vi "Parameter.vi"(8 "error in":errorcluster, 11 "Node Ptr":T1 format="%.0x") -> (0 "error out":errorcluster)   [LabVIEW 2020, in "Ballard MIL-STD-1553 System Explorer.lvlib" / "Implementation.lvlib"]
uses:
  Implementation.lvlib
  <vilib>/NI VeriStand/Custom Device API/Custom Device Item Ref.ctl
  <vilib>/NI VeriStand/Custom Device API/Custom Device API.lvlib
  Scripting/Ballard MIL-STD-1553 Scripting.lvlib
panel:
  out "Encoding Type":enum16{"BNR", "BCD", "Discrete"}(ring)
  out "Unit":string
  out "Scale Offset":dbl
  out "Scale Factor":dbl=1.0
  out "Signed?":bool=TRUE
  out "Number of Bits":i32=16
  out "Start Bit":i32
  out "default value":dbl caption="Default Value (Scaled)"
  in  "SHDocVw.IWebBrowser":refnum<k7>(container)
  in  "General Header":cluster{"Section Name":string}={"Section Name"="Ballard MIL-STD-1553 - Parameter"}
  in  "Description":string
  out "Name":string
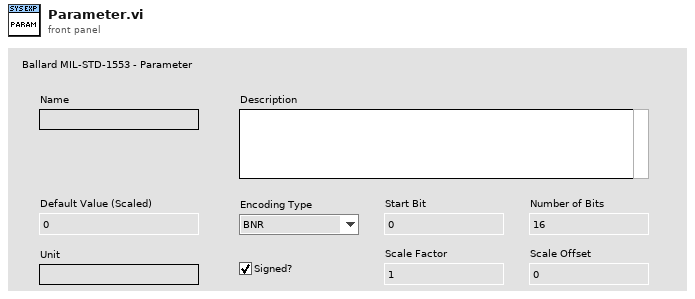
[diagram p1: front panel]
types:
  T1 = typedef "Custom Device API.lvlib/Custom Device Item Ref.ctl" = u64
  T2 = typedef "Custom Device API.lvlib/Custom Device Channel.ctl" = cluster{"Type":T3, "Units":string, "Default Value":dbl, "Faultable":bool, "Scalable":bool}
  T3 = typedef "Custom Device API.lvlib/Custom Device Channel Type.ctl" = enum16{"Input", "Output"}
  T4 = typedef "Parameter Definition.ctl" = cluster{"start index":i32, "size (bits)":i32, "encoding":enum16{"BNR", "BCD", "Discrete"}, "signed":bool, "multiplier":dbl, "offset":dbl}
  T5 = typedef "Custom Device API.lvlib/Custom Device Commands.ctl" = enum16{"Default", "Item renamed", "Shutdown", "Dynamic button pressed"}
  T6 = typedef "Custom Device API.lvlib/Custom Device Item Info.ctl" = cluster{"Name":string, "Is Channel":bool, "GUID":string, "Is Waveform":bool}
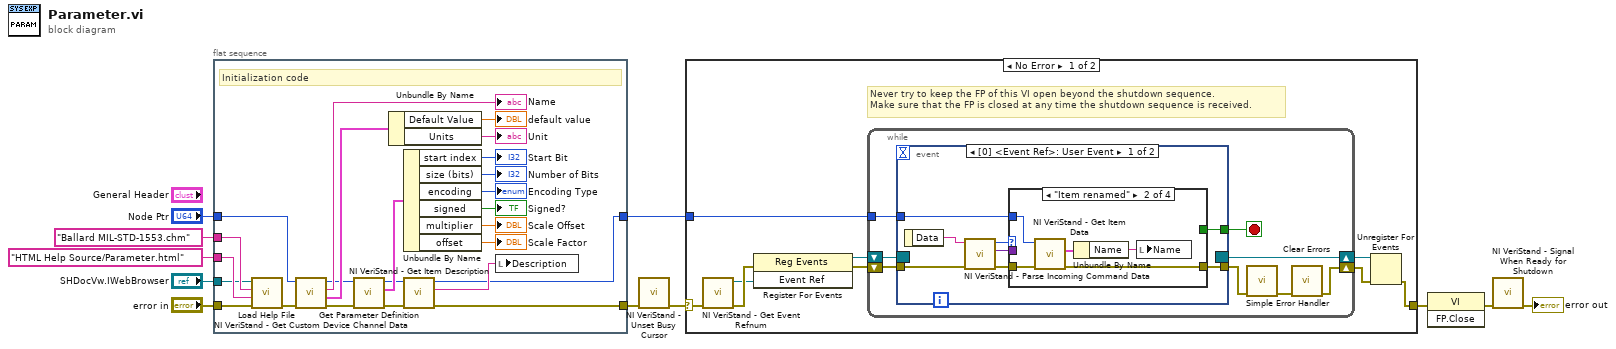
[diagram p0: block diagram]
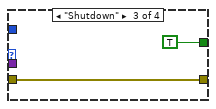
[diagram p3: hidden frame]
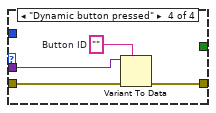
[diagram p4: hidden frame]
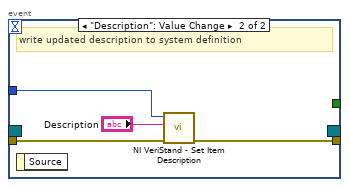
[diagram p5: hidden frame]
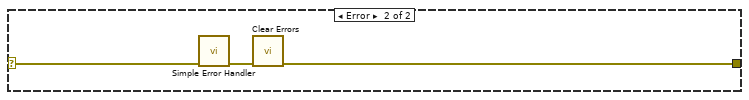
[diagram p6: hidden frame]
diagram:
  n1 = flat-sequence "Initialization code" {
    tunnel: "error in" -> [w34]
    tunnel: "Node Ptr" -> [w30]
    tunnel: [w13] -> w7
    tunnel: [w12] -> w4
    tunnel: "SHDocVw.IWebBrowser" -> [w31]
    tunnel: "HTML Help Source/Parameter.html" ("CD_CHM_Section") -> [w33]
    tunnel: "Ballard MIL-STD-1553.chm" ("CD_CHM_FileName") -> [w32]
    frame #0 {
      # "Initialization code"
      n2 = call "Load Help File.vi"("error in (no error)"=w34, "HTML File to Load"=w33, "Main CHM File"=w32, "Browser"=w31) -> ("error out"=w28:errorcluster)  [unwired: 7 in]
      n3 = call <vilib>:"NI VeriStand - Get Custom Device Channel Data.vi"("error in (no error)"=w28, "Channel Ref in"=w30) -> ("error out"=w16:errorcluster, "Channel"=w29:T2, "Channel Name"=→"Name":string, "Channel Ref out"=w17:T1)  [unwired: 4 in, 2 out]
      n4 = call "Get Parameter Definition.vi"("error in"=w16, "parameter in"=w17) -> ("error out"=w14:errorcluster, "parameter definition"=w24:T4, "parameter out"=w15:T1)  [unwired: 7 in]
      n5 = Unbundle By Name(w29) -> ("Default Value"=→"default value":dbl, "Units"=→"Unit":string)
      n6 = Unbundle By Name(w24) -> ("start index"=→"Start Bit":i32, "size (bits)"=→"Number of Bits":i32, "encoding"=→"Encoding Type":enum16{"BNR", "BCD", "Discrete"}, "signed"=→"Signed?":bool, "multiplier"=→"Scale Offset":dbl, "offset"=→"Scale Factor":dbl)
      n7 = call <vilib>:"NI VeriStand - Get Item Description.vi"("error in (no error)"=w14, "Item Ref in"=w15) -> ("error out"=w13:errorcluster, "Description"=w35:string, "Item Ref out"=w12:T1)  [unwired: 7 out]
      n8 = local write "Description"(w35) -> ()
    }
  }
  n9 = call <vilib>:"NI VeriStand - Unset Busy Cursor.vi"("error in (no error)"=w7) -> ("error out"=w6:errorcluster)  [unwired: 10 out]
  n10 = case shown="No Error" w6 {
    selector: w6 -> [w36 w79]
    tunnel: [w41 w77] -> w11
    tunnel: w4 -> [w37 _]
    frame No Error {
      # "Never try to keep the FP of this VI open beyond the shutdown sequence.\nMake sure that the FP is closed at any time the shutdown sequence is received."
      n11 = call <vilib>:"NI VeriStand - Get Event Refnum.vi"("error in (no error)"=w36) -> ("error out"=w44:errorcluster, "Event Ref"=w40:refnum<user-event>)  [unwired: 9 out]
      n12 = register-events(error in=w44, w40) -> (reference out=w38:refnum<event-registration>, error out=w39:errorcluster)  [unwired: 1 in]
      n13 = while {
        tunnel: w37 -> [w48]
        shift-right: [w45] -> w42
        shift-left: w39 -> [w51]
        shift-right: [w52] -> w43
        shift-left: w38 -> [w50]
        stop <- w49 stop-if-true
        n14 = event shown="[0] <Event Ref>: User Event" {
          selector: w50 -> [_ _]
          dyn-events: [_ _] -> w52
          timeout: _ -> [_ _]
          tunnel: w51 -> [w60 w75]
          tunnel: [w57 _] -> w49
          tunnel: [w56 w74] -> w47
          tunnel: w48 -> [w55 w76]
          event User Event {
            n15 = event-data() -> ("Data"=w53:string)  [unwired: 1 out]
            n16 = call <vilib>:"NI VeriStand - Parse Incoming Command Data.vi"("error in (no error)"=w60, "Incoming data"=w53) -> ("error out"=w59:errorcluster, "Outgoing data"=w54:variant, "Action"=w58:T5)  [unwired: 7 out]
            n17 = case shown="\"Item renamed\"" w58 {
              tunnel: w59 -> [w61 w66 w67 w72]
              tunnel: [_ _ TRUE _] -> w57
              tunnel: [w61 w63 w67 w69] -> w56
              tunnel: w55 -> [_ w65 _ _]
              tunnel: w54 -> [_ _ _ w71]
              frame Default {
              }
              frame "Item renamed" {
                n18 = call <vilib>:"NI VeriStand - Get Item Data.vi"("error in (no error)"=w66, "Item Ref in"=w65) -> ("error out"=w63:errorcluster, "Item Info"=w64:T6)  [unwired: 8 out]
                n19 = Unbundle By Name(w64) -> ("Name"=w62:string)
                n20 = local write "Name"(w62) -> ()
              }
              frame "Shutdown" {
              }
              frame "Dynamic button pressed" {
                w70 = ""  # Button ID
                n21 = Variant To Data(error in=w72, type=w70, Variant=w71) -> (error out=w69:errorcluster)  [unwired: 1 out]
              }
            }
          }
          event "Description": Value Change {
            # "write updated description to system definition"
            n22 = event-data() -> ()  [unwired: 2 out]
            n23 = call <vilib>:"NI VeriStand - Set Item Description.vi"("error in (no error)"=w75, "Description"="Description", "Item Ref in"=w76) -> ("error out"=w74:errorcluster)  [unwired: 8 out]
          }
        }
        n24 = call <vilib>:"Simple Error Handler.vi"("error in (no error)"=w47) -> ("error out"=w46:errorcluster)  [unwired: 1 in, 7 out]
        n25 = call <vilib>:"Clear Errors.vi"("error in (no error)"=w46) -> ("error out"=w45:errorcluster)  [unwired: 1 in, 5 out]
      }
      n26 = Unregister For Events(event registration refnum=w43, error in=w42) -> (error out=w41:errorcluster)
    }
    frame Error {
      n27 = call <vilib>:"Simple Error Handler.vi"("error in (no error)"=w79) -> ("error out"=w78:errorcluster)  [unwired: 1 in, 7 out]
      n28 = call <vilib>:"Clear Errors.vi"("error in (no error)"=w78) -> ("error out"=w77:errorcluster)  [unwired: 1 in, 5 out]
    }
  }
  n29 = invoke class="VI" method="FP.Close"(error in=w11) -> (error out=w10:errorcluster)  [unwired: 2 in, 2 out]
  n30 = call <vilib>:"NI VeriStand - Signal When Ready for Shutdown.vi"("error in (no error)"=w10) -> ("error out"=→"error out":errorcluster)  [unwired: 10 out]
